vi "recalc_drift.vi"(8 "error in (no error)":errorcluster caption="错误输入（无错误）", 11 "MotorSystem 输入":refnum<class "MotorSystem.lvclass">) -> (0 "error out":errorcluster caption="错误输出", 3 "MotorSystem 输出":refnum<class "MotorSystem.lvclass">)   [LabVIEW 2014, in "MotorSystem.lvclass"]
uses:
  MotorSystem.lvclass
  OneMotion/OneMotion.lvclass
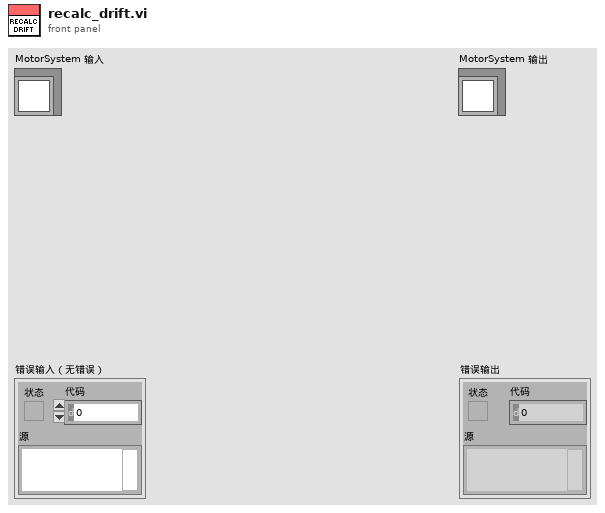
[diagram p1: front panel]
types:
  T1 = typedef "MotorSystem.lvclass/MotionCluster.ctl" = cluster{"OneMotion.lvclass":refnum<class "OneMotion.lvclass">, "connected?":bool, "default enabled?":bool, "enabled?":bool}
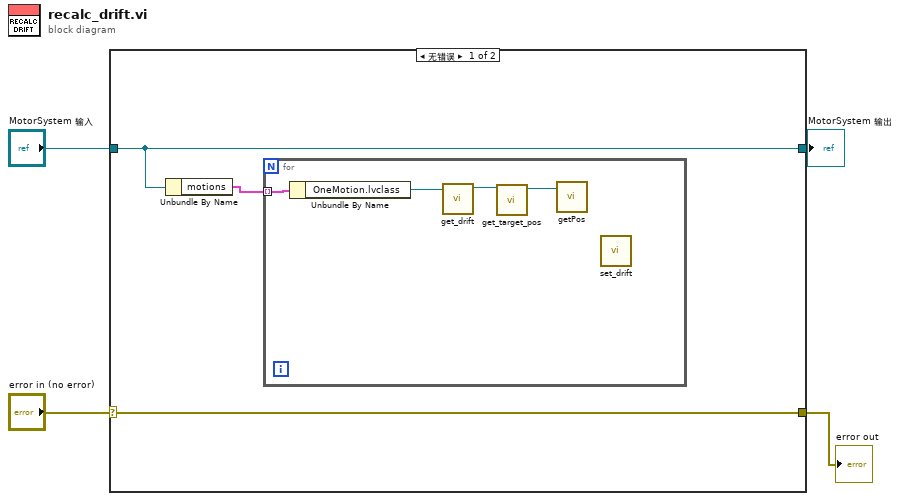
[diagram p0: block diagram]
diagram:
  n1 = case shown="无错误" "error in (no error)" {
    selector: "error in (no error)" -> [w7 w13]
    tunnel: [w7 w13] -> w3
    tunnel: [w6 w12] -> w1
    tunnel: "MotorSystem 输入" -> [w6 w12]
    frame No Error {
      n2 = Unbundle By Name(w6) -> ("motions"=w5:T1[])
      n3 = for {
        tunnel: w5 -> [w11] mode=indexing
        n4 = Unbundle By Name(w11) -> ("OneMotion.lvclass"=w10:refnum<class "OneMotion.lvclass">)
        n5 = call "get_drift.vi"("OneMotion输入"=w10) -> ("OneMotion输出"=w9:refnum<class "OneMotion.lvclass">)  [unwired: 8 in, 2 out]
        n6 = call "get_target_pos.vi"("OneMotion输入"=w9) -> ("OneMotion输出"=w8:refnum<class "OneMotion.lvclass">)  [unwired: 8 in, 2 out]
        n7 = call "getPos.vi"("OneMotion 输入"=w8) -> ()  [unwired: 8 in, 3 out]
        n8 = call "set_drift.vi"() -> ()  [unwired: 10 in, 2 out]
      }
    }
    frame Error {
    }
  }
  "error out" <- w3
  "MotorSystem 输出" <- w1
